vi "Close Logger.vi"(8 "error in (no error)":errorcluster, 11 "Logger in":refnum<class "Logger.lvclass">) -> (0 "error out":errorcluster)   [LabVIEW 2020, in "LV Log.lvlib" / "Logger.lvclass"]
uses:
  Logger.lvclass
  Logger.lvclass/Logger.ctl
  Sinks/Sink/Sink.lvclass
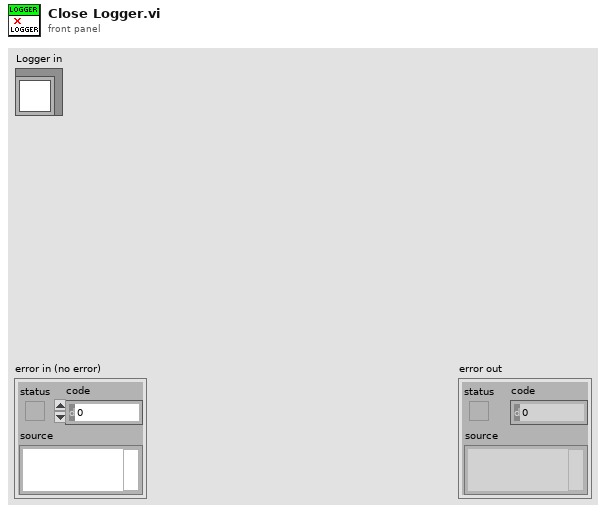
[diagram p1: front panel]
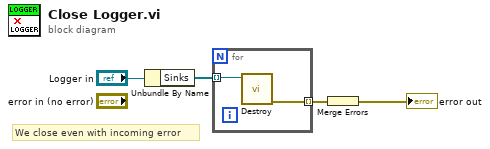
[diagram p0: block diagram]
diagram:
  # "We close even with incoming error"
  n1 = Unbundle By Name("Logger in") -> ("Sinks"=w2:refnum<class "Sink.lvclass">[])
  n2 = for {
    tunnel: w2 -> [w6] mode=indexing
    tunnel: [w5] -> w1 mode=indexing
    n3 = call-dynamic "Destroy.vi"("Sink in"=w6) -> ("error out"=w5:errorcluster)  [unwired: 9 in, 1 out]
  }
  n4 = Merge Errors(w1) -> (→"error out":errorcluster)
